vi "BPSK.vi"() -> ()   [LabVIEW 2012]
panel:
  out "Demodulated PSK":dynamicdata(graph)
  out "Waveform Graph 3":dynamicdata(graph)
  out "BPSK":dynamicdata(graph)
  out "Binary Data":dynamicdata(graph) caption="Square"
  in  "Slide 2":dbl(slide) scale=0.0..500.0
  in  "Slide":dbl(slide) scale=0.0..5000.0
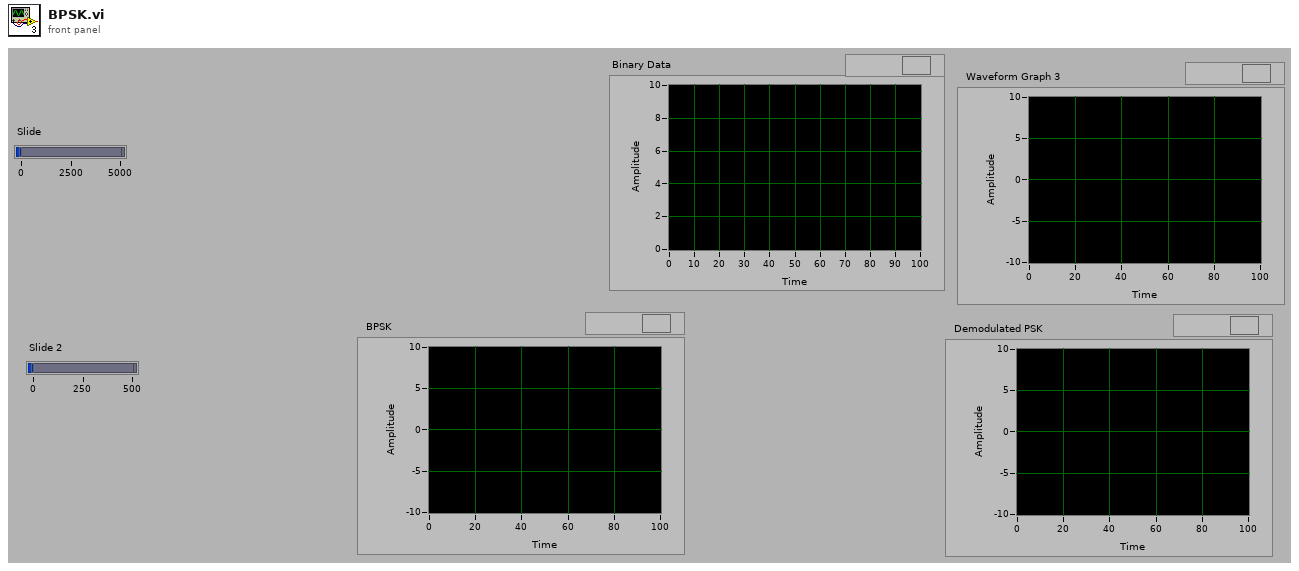
[diagram p1: front panel]
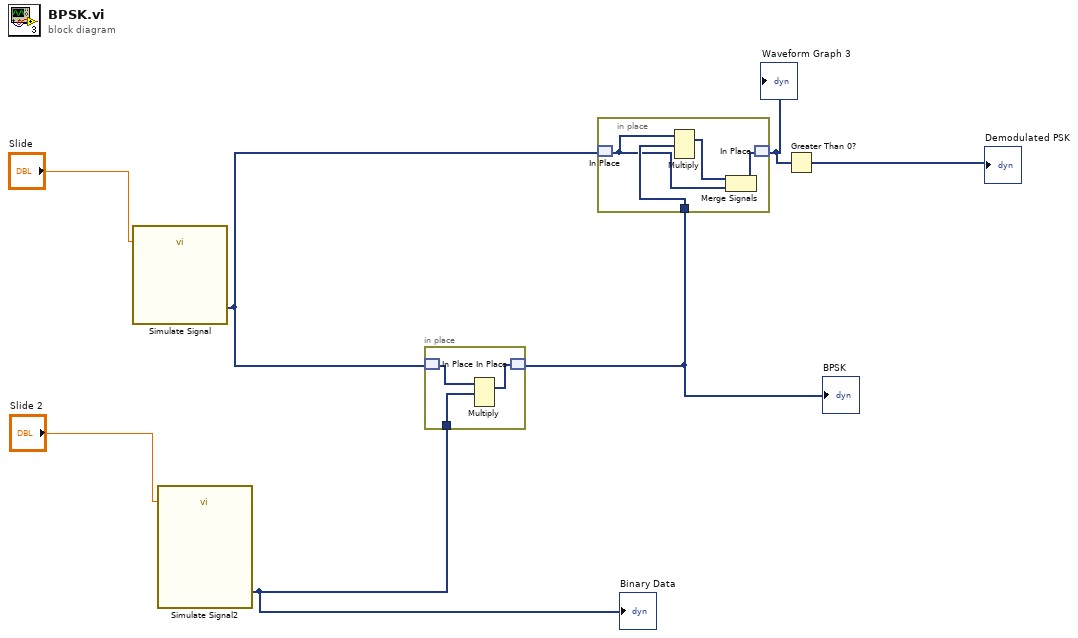
[diagram p0: block diagram]
diagram:
  n1 = call "Simulate Signal"("Frequency"="Slide") -> ("Sine"=w4:dynamicdata)  [unwired: 13 in, 1 out]
  n2 = call "Simulate Signal2"("Frequency"="Slide 2") -> ("Square"=w5:dynamicdata)  [unwired: 13 in, 1 out]
  "Binary Data" <- w5
  n3 = in-place {
    in-place-border: w5 -> [w10]
    n4 = in-place-match #1(w4) -> (w9:dynamicdata)
    n5 = Multiply(1:w10, 2:w9) -> (0:w8:dynamicdata)  [unwired: 1 in, 1 out]
    n6 = in-place-match #1(w8) -> (w3:dynamicdata)
  }
  "BPSK" <- w3
  n7 = in-place {
    in-place-border: w3 -> [w14]
    n8 = in-place-match #2(w4) -> (w11:dynamicdata)
    n9 = Multiply(1:w14, 2:w11) -> (0:w13:dynamicdata)  [unwired: 1 in, 1 out]
    n10 = Merge Signals(w13, w11) -> (w12:dynamicdata)
    n11 = in-place-match #2(w12) -> (w2:dynamicdata)
  }
  "Waveform Graph 3" <- w2
  n12 = Greater Than 0?(x=w2) -> (x > 0?=→"Demodulated PSK":dynamicdata)
